vi "Multiple Target Analysis.vi"(6 "gun tracking mode":T1, 8 "Image Size":cluster{i32, i32}, 9 "Camera Type":enum16{"206", "1011"}(ring), 10 "Score Limits":T10={"Rect Coverage"=70.0, "Aspect Ratio"=0.0, "X Edge Strength"=40.0, "Y Edge Strength"=50.0}, 11 "Targets":T11[](array[typedef])) -> (1 "Targetting Output":T3, 2 "Diamond Targets":T4[](array[typedef]), 3 "Lines":T7[][](array[typedef]))   [LabVIEW 2011]
uses:
  Target Data.ctl
  Line.ctl
  Direction.ctl
  Line Confidence.ctl
  Diamond Target Output.ctl
  Rectangle Position.ctl
  Target Confidence.ctl
  Camera State.ctl
  gun/gun_tracking_mode.ctl
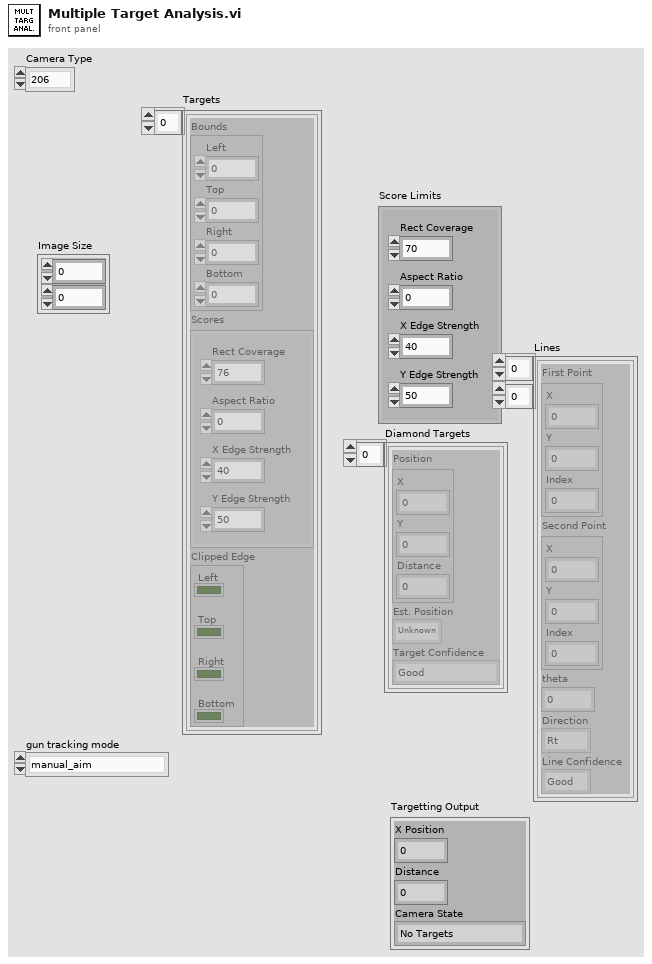
[diagram p1: front panel]
types:
  T1 = typedef "gun_tracking_mode.ctl" = enum16{"manual_aim", "auto_aim_camera", "preset_center_field", "preset_right_pocket", "preset_left_pocket", "align_center", "align_center_backwards", "auto_aim_key", "align_fold", "auton_custom", "preset_pass", "auto_aim_auton"}
  T2 = typedef "Camera State.ctl" = enum16{"No Targets", "Low Confidence", "Medium Confidence", "High Confidence", "Camera Error"}
  T3 = cluster{"X Position":dbl, "Distance":dbl, "Camera State":T2}
  T4 = typedef "Diamond Target Output.ctl" = cluster{"Position":cluster{"X":dbl, "Y":dbl, "Distance":dbl}, "Est. Position":T5, "Target Confidence":T6}
  T5 = typedef "Rectangle Position.ctl" = enum16{"Unknown", "Top", "Right", "Left", "Bottom"}
  T6 = typedef "Target Confidence.ctl" = enum16{"Good", "Good-Clipped Y", "Marginal-Clipped X"}
  T7 = typedef "Line.ctl" = cluster{"First Point":cluster{"X":dbl, "Y":dbl, "Index":dbl}, "Second Point":cluster{"X":dbl, "Y":dbl, "Index":dbl}, "theta":dbl, "Direction":T8, "Line Confidence":T9}
  T8 = typedef "Direction.ctl" = enum16{"Rt", "Rt-Up", "Up", "Lt-Up", "Lt", "Lt-Dn", "Dn", "Rt-Dn", "Unknown"}
  T9 = typedef "Line Confidence.ctl" = enum16{"Good", "Bad"}
  T10 = cluster{"Rect Coverage":dbl, "Aspect Ratio":dbl, "X Edge Strength":dbl, "Y Edge Strength":dbl}
  T11 = typedef "Target Data.ctl" = cluster{"Bounds":cluster{"Left":dbl, "Top":dbl, "Right":dbl, "Bottom":dbl}, "Scores":cluster{"Rect Coverage":dbl, "Aspect Ratio":dbl, "X Edge Strength":dbl, "Y Edge Strength":dbl}, "Clipped Edge":cluster{"Left":bool, "Top":bool, "Right":bool, "Bottom":bool}}
  T12 = typedef "Target.ctl" = cluster{"Target Center":cluster{"X":dbl, "Y":dbl}, "Distance (ft)":dbl, "Bounds":cluster{"Left":dbl, "Top":dbl, "Right":dbl, "Bottom":dbl}, "Clipped Edge":cluster{"Left":bool, "Top":bool, "Right":bool, "Bottom":bool}}
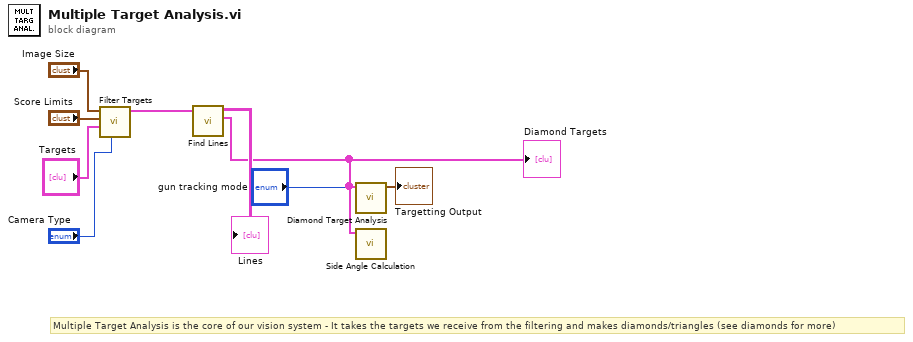
[diagram p0: block diagram]
diagram:
  # "Multiple Target Analysis is the core of our vision system - It takes the targets we receive from the filtering and makes diamonds/triangles (see diamonds for more)"
  n1 = call "Filter Targets.vi"("Camera Type"="Camera Type", "Targets"="Targets", "Score Limits"="Score Limits", "Image Size"="Image Size") -> ("Filtered Targets"=w4:T12[])  [unwired: 7 in]
  n2 = call "Find Lines.vi"("Filtered Targets"=w4) -> ("Diamond Targets"=w2:T4[], "Lines"=→"Lines":T7[][])  [unwired: 9 in]
  "Diamond Targets" <- w2
  n3 = call "Diamond Target Analysis.vi"("gun tracking mode"="gun tracking mode", "Diamond Targets"=w2) -> ("Targetting Output"=→"Targetting Output":T3)  [unwired: 9 in]
  n4 = call "Side Angle Calculation.vi"("Diamond Targets"=w2) -> ()  [unwired: 10 in, 1 out]
